vi "Elapsed time(ms).vi"(10 "Target":u32) -> (1 "Elapsed Time":u32, 2 "Elapsed ?":bool)   [LabVIEW 2017]
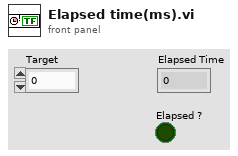
[diagram p1: front panel]
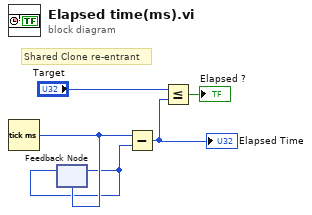
[diagram p0: block diagram]
diagram:
  # "Shared Clone re-entrant"
  n1 = Tick Count (ms)() -> (millisecond timer value=w2:u32)
  n2 = feedback #1(w2) -> (w1:u32)
  n3 = feedback-in #1(w1) -> ()
  n4 = Subtract(x=w2, y=w1) -> (x-y=w3:u32)
  "Elapsed Time" <- w3
  n5 = Less Or Equal?(x="Target", y=w3) -> (x <= y?=→"Elapsed ?":bool)
